vi "HoloPy_subvolume_3planes.vi"(8 "error in (no error)":errorcluster, 10 "param":T1, 11 "Refnum in":refnum<k35>) -> (0 "error out":errorcluster, 2 "YZ Plane":sgl[][](array[numeric]), 3 "Refnum out":refnum<k35>)   [LabVIEW 2025, in "holoTracker.lvlib"]
uses:
  holoTracker.lvlib
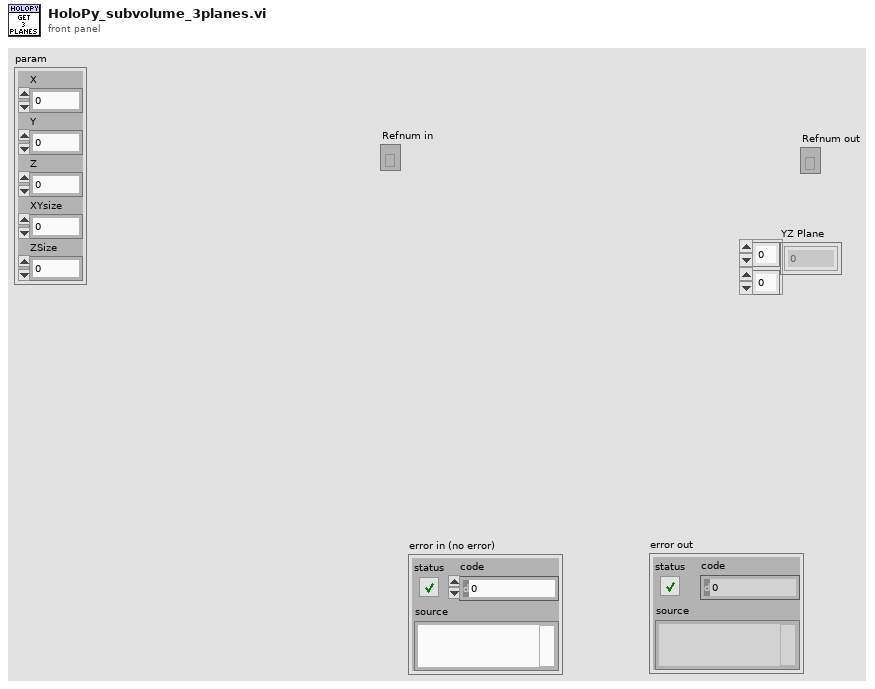
[diagram p1: front panel]
types:
  T1 = cluster{"X":i32, "Y":i32, "Z":i32, "XYsize":i32, "ZSize":i32}
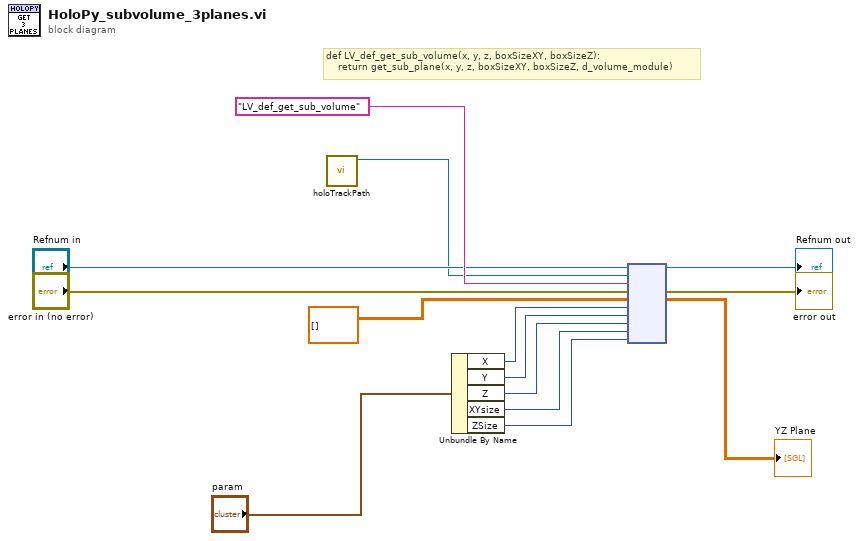
[diagram p0: block diagram]
diagram:
  # "def LV_def_get_sub_volume(x, y, z, boxSizeXY, boxSizeZ):\n    return get_sub_plane(x, y, z, boxSizeXY, boxSizeZ, d_volume_module)"
  n1 = call "holoTrackPath.vi"() -> ("appended path"=w7:path)  [unwired: 11 in]
  n2 = Unbundle By Name("param") -> ("X"=w5:i32, "Y"=w4:i32, "Z"=w3:i32, "XYsize"=w2:i32, "ZSize"=w1:i32)
  n3 = node("Refnum in", w7, "LV_def_get_sub_volume" ("function name"), "error in (no error)", sgl[][] [], w5, w4, w3, w2, w1) -> (→"Refnum out":refnum<k35>, →"error out":errorcluster, →"YZ Plane":sgl[][])  [unwired: 5 in, 2 out]
